vi "Get Magnet ID.vi"() -> (0 "String":string)   [LabVIEW 2020]
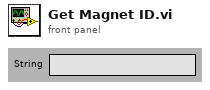
[diagram p1: front panel]
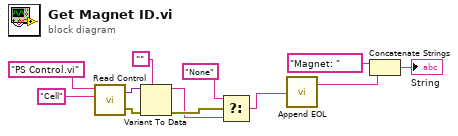
[diagram p0: block diagram]
diagram:
  n1 = call "Read Control.vi"("VI Name"="PS Control.vi", "Control Name"="Cell") -> ("Value"=w9:variant, "error out"=w5:errorcluster)  [unwired: 3 in]
  n2 = Variant To Data(error in=w5, type="", Variant=w9) -> (data=w3:string, error out=w4:errorcluster)
  n3 = Select(t="None", s=w4, f=w3) -> (s? t:f=w2:string)
  n4 = call "Append EOL.vi"("INPUT STRING"=w2) -> ("OUTPUT STRING (PLUS End of Line)"=w12:string)
  n5 = Concatenate Strings("Magnet: ", w12) -> (→"String":string)
